vi "Prog_Revision_Date.vi"(5 "Input string":string) -> (0 "Revision time (s)":u32, 2 "svnBaseRevision":u32, 3 "Prog's last revision date":string)   [LabVIEW 2020]
uses:
  <vilib>/Utility/miscctls.llb/LVDateTimeRec.ctl
panel:
  out "source":string
  out "Prog's last revision time":string
  out "RevisionData":string
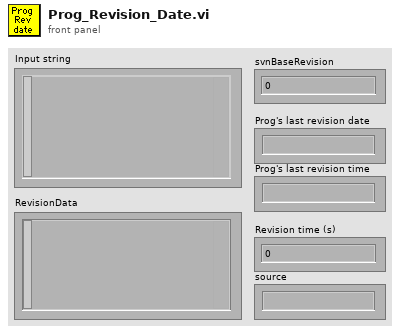
[diagram p1: front panel]
types:
  T1 = typedef "LVDateTimeRec.ctl" = cluster{"fractional second":dbl, "second":i32, "minute":i32, "hour":i32, "day of month":i32, "month":i32, "year":i32, "day of week":i32, "day of year":i32, "DST":i32}
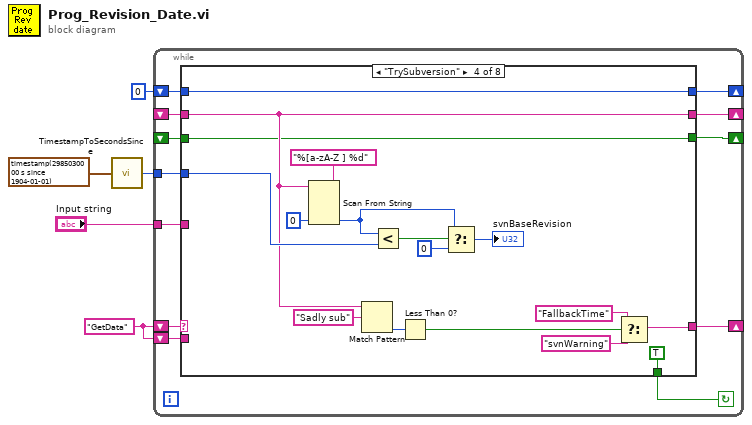
[diagram p0: block diagram]
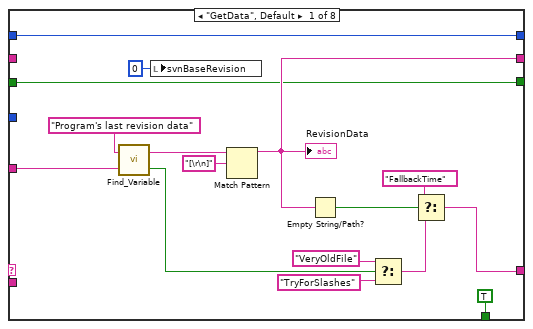
[diagram p2: hidden frame]
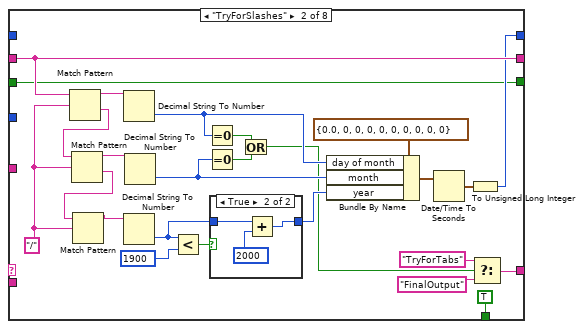
[diagram p3: hidden frame]
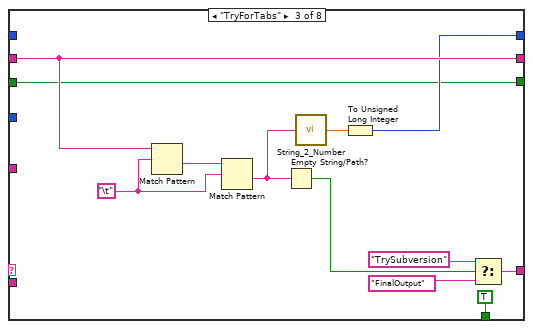
[diagram p5: hidden frame]
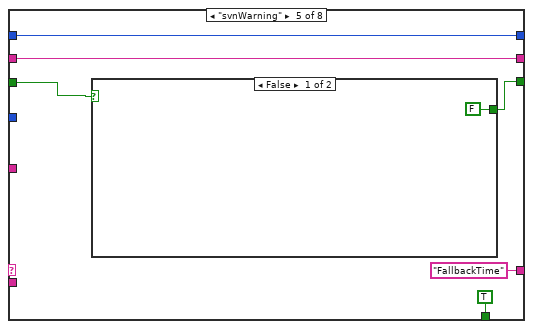
[diagram p6: hidden frame]
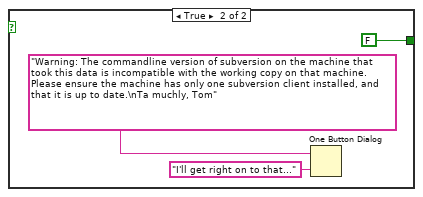
[diagram p7: hidden frame]
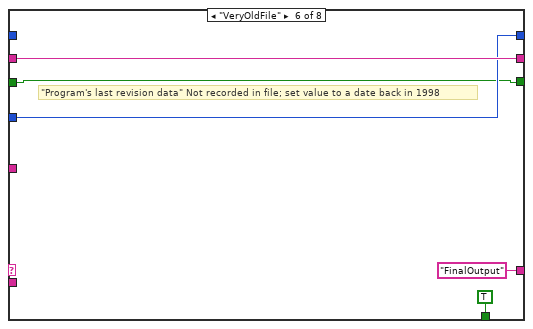
[diagram p8: hidden frame]
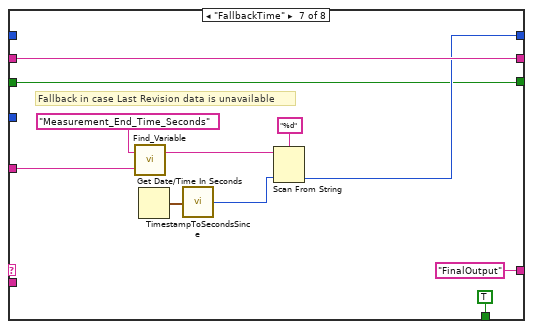
[diagram p9: hidden frame]
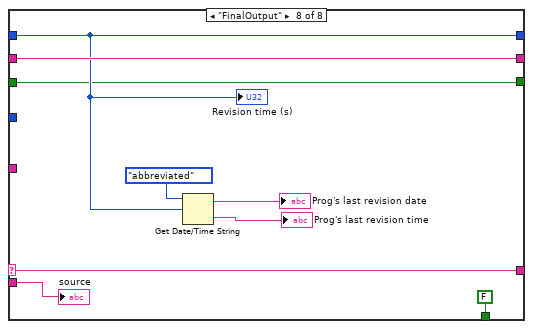
[diagram p10: hidden frame]
diagram:
  w1 = "GetData"
  n1 = call "TimestampToSecondsSince.vi"("Time Stamp Control"=timestamp(2985030000 s since 1904-01-01)) -> ("unsigned 32bit integer"=w2:u32)
  n2 = while {
    tunnel: "Input string" -> [w17]
    shift-right: [w15] -> _
    shift-left: w1 -> [w16]
    shift-right: [w14] -> _
    shift-left: u32 0 -> [w13]
    shift-right: [w11] -> _
    shift-left: _ -> [w10]
    tunnel: w2 -> [w9]
    shift-left: w1 -> [w8]
    shift-right: [w6] -> _
    shift-left: _ -> [w7]
    stop <- w12 continue-if-true
    n3 = case shown="\"TrySubversion\"" w16 {
      selector: w16 -> [_ _ _ _ _ _ _ w120]
      tunnel: w17 -> [w30 _ _ _ _ _ w113 _]
      tunnel: [w21 w42 w71 w81 "FallbackTime" ("t") "FinalOutput" "FinalOutput" w120] -> w15
      tunnel: [w27 w44 w65 w91 w97 w103 w110 w122] -> w14
      tunnel: w13 -> [w27 _ _ w91 w97 _ _ w122]
      tunnel: [TRUE TRUE TRUE TRUE TRUE TRUE TRUE FALSE] -> w12
      tunnel: [w24 w45 w72 w84 w96 w104 w117 w126] -> w11
      tunnel: w10 -> [_ w45 w72 w84 w96 w104 w117 w126]
      tunnel: w9 -> [_ _ _ w88 _ w103 _ _]
      tunnel: w8 -> [_ _ _ _ _ _ _ w119]
      tunnel: w7 -> [w18 w34 w63 w77 w93 w102 w107 w118]
      tunnel: [w18 w34 w63 w77 w92 w102 w107 w118] -> w6
      frame "GetData", Default {
        n4 = call "Find_Variable.vi"("Input string"=w30, "Variable name"="Program's last revision data") -> ("No Match?"=w29:bool, "After  Matched string"=w32:string)
        n5 = local write "svnBaseRevision"(0 ("svnBaseRevision")) -> ()
        n6 = Match Pattern(string=w32, regular expression="[\r\n]") -> (before substring=w24:string)  [unwired: 4 out]
        "RevisionData" <- w24
        n7 = Empty String/Path?(string/path=w24) -> (empty?=w22:bool)
        n8 = Select(t="VeryOldFile", s=w29, f="TryForSlashes") -> (s? t:f=w23:string)
        n9 = Select(t="FallbackTime", s=w22, f=w23) -> (s? t:f=w21:string)
      }
      frame "TryForSlashes" {
        w46 = "/" ("search char (-)")
        n10 = Match Pattern(string=w45, regular expression=w46) -> (before substring=w47:string, after substring=w48:string)  [unwired: 3 out]
        n11 = Match Pattern(string=w48, regular expression=w46) -> (before substring=w49:string, after substring=w51:string)  [unwired: 3 out]
        n12 = Match Pattern(string=w51, regular expression=w46) -> (before substring=w50:string)  [unwired: 4 out]
        n13 = Decimal String To Number(string=w47) -> (number=w39:i32)  [unwired: 3 out]
        n14 = Decimal String To Number(string=w50) -> (number=w55:i32)  [unwired: 3 out]
        n15 = Decimal String To Number(string=w49) -> (number=w38:i32)  [unwired: 3 out]
        n16 = Less?(x=w55, y=1900) -> (x < y?=w54:bool)
        n17 = Equal To 0?(x=w39) -> (x = 0?=w37:bool)
        n18 = Equal To 0?(x=w38) -> (x = 0?=w36:bool)
        n19 = case shown="True" w54 {
          tunnel: w55 -> [w59 w61]
          tunnel: [w59 w60] -> w56
          frame False {
          }
          frame True {
            n20 = Add(x=w61, y=2000) -> (x+y=w60:i32)
          }
        }
        n21 = Or(x=w37, y=w36) -> (x .or. y?=w35:bool)
        n22 = Bundle By Name(cluster=T1 {"fractional second"=0.0, "second"=0, "minute"=0, "hour"=0, "day of month"=0, "month"=0, "year"=0, "day of week"=0, "day of year"=0, "DST"=0} ("date time rec"), "day of month"=w39, "month"=w38, "year"=w56) -> (w58:T1)
        n23 = Date/Time To Seconds(2:w58) -> (0:w52:timestamp)  [unwired: 1 in]
        n24 = To Unsigned Long Integer(number=w52) -> (unsigned 32bit integer=w44:u32)
        n25 = Select(t="TryForTabs", s=w35, f="FinalOutput") -> (s? t:f=w42:string)
      }
      frame "TryForTabs" {
        w74 = "\t"
        n26 = Match Pattern(string=w72, regular expression=w74) -> (after substring=w73:string)  [unwired: 4 out]
        n27 = Match Pattern(string=w73, regular expression=w74) -> (after substring=w66:string)  [unwired: 4 out]
        n28 = Empty String/Path?(string/path=w66) -> (empty?=w70:bool)
        n29 = call "String_2_Number.vi"("Value"=w66) -> ("Numeric"=w67:dbl)
        n30 = To Unsigned Long Integer(number=w67) -> (unsigned 32bit integer=w65:u32)
        n31 = Select(t="TrySubversion", s=w70, f="FinalOutput") -> (s? t:f=w71:string)
      }
      frame "TrySubversion" {
        n32 = Scan From String(format string="%[a-zA-Z ] %d", input string=w84, default 2=u32 0 ("unsigned 32bit integer")) -> (output 2=w76:u32)  [unwired: 4 in, 3 out]
        n33 = Match Pattern(string=w84, regular expression="Sadly sub") -> (offset past match=w82:i32)  [unwired: 1 in, 3 out]
        n34 = Less?(x=w76, y=w88) -> (x < y?=w87:bool)
        n35 = Less Than 0?(x=w82) -> (x < 0?=w79:bool)
        n36 = Select(t=w76, s=w87, f=u32 0) -> (s? t:f=→"svnBaseRevision":u32)
        n37 = Select(t="FallbackTime", s=w79, f="svnWarning" ("t")) -> (s? t:f=w81:string)
      }
      frame "svnWarning" {
        n38 = case shown="False" w93 {
          tunnel: [FALSE FALSE] -> w92
          frame False {
          }
          frame True {
            n39 = One Button Dialog(message="Warning: The commandline version of subversion on the machine that took this data is incompatible with the working copy on that machine. Please ensure the machine has only one subversion client installed, and that it is up to date.\nTa muchly, Tom", button name ("OK")="I'll get right on to that...") -> ()  [unwired: 1 out]
          }
        }
      }
      frame "VeryOldFile" {
        # "\"Program's last revision data\" Not recorded in file; set value to a date back in 1998"
      }
      frame "FallbackTime" {
        # "Fallback in case Last Revision data is unavailable"
        n40 = call "Find_Variable.vi"("Input string"=w113, "Variable name"="Measurement_End_Time_Seconds") -> ("After  Matched string"=w114:string)  [unwired: 1 out]
        n41 = Get Date/Time In Seconds() -> (seconds since 1Jan1904=w109:timestamp)
        n42 = call "TimestampToSecondsSince.vi"("Time Stamp Control"=w109) -> ("unsigned 32bit integer"=w108:u32)
        n43 = Scan From String(format string="%d", input string=w114, default 1=w108) -> (output 1=w110:u32)  [unwired: 2 in, 3 out]
      }
      frame "FinalOutput" {
        n44 = Get Date/Time String(date format (0)=enum16{"short", "long", "abbreviated"}."abbreviated", seconds (now)=w122) -> (date string=→"Prog's last revision date":string, time string=→"Prog's last revision time":string)  [unwired: 1 out]
        "Revision time (s)" <- w122
        "source" <- w119
      }
    }
  }
